vi "Update Steps LEDs.vi"(8 "error in":errorcluster, 10 "Wash Steps Selected":T1(array[cluster]), 11 "Car Wash Indicators Ref":refnum<vi>) -> (0 "error out":errorcluster)   [LabVIEW 2020]
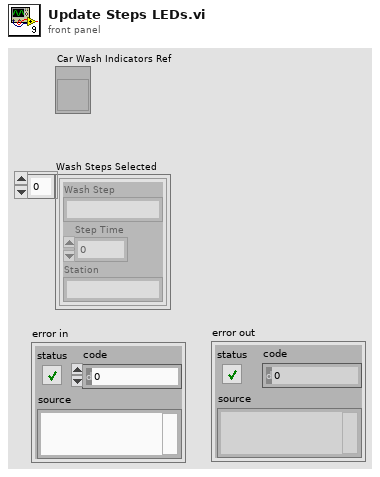
[diagram p1: front panel]
types:
  T1 = cluster{"Wash Step":string, "Step Time":i32, "Station":string}[]
  T2 = cluster{"Wash Step":string, "Step Time":i32, "Station":string}
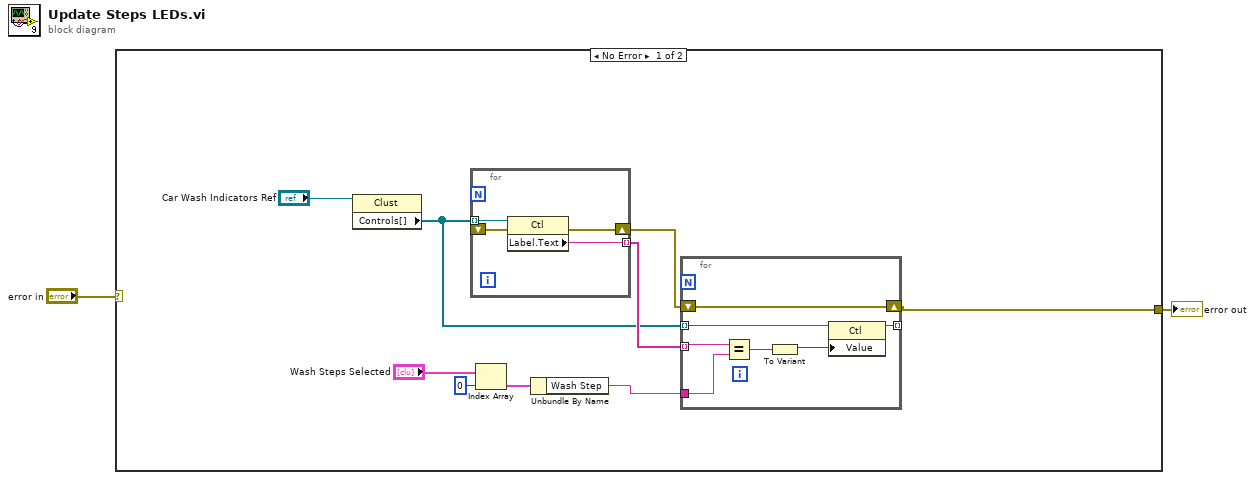
[diagram p0: block diagram]
diagram:
  n1 = case shown="No Error" "error in" {
    selector: "error in" -> [_ w23]
    tunnel: [w3 w23] -> w2
    frame No Error {
      n2 = property class="Clust"(reference="Car Wash Indicators Ref") -> ("Controls[]"=w5:refnum<vi>[])  [unwired: 1 in, 2 out]
      n3 = for {
        tunnel: w5 -> [w22] mode=indexing
        tunnel: [w21] -> w7 mode=indexing
        shift-right: [w20] -> w6
        shift-left: _ -> [w19]
        n4 = property class="Ctl"(reference=w22, error in=w19) -> (error out=w20:errorcluster, "Label.Text"=w21:string)  [unwired: 1 out]
      }
      n5 = Index Array(array="Wash Steps Selected", index=0) -> (element=w10:T2)
      n6 = Unbundle By Name(w10) -> ("Wash Step"=w11:string)
      n7 = for {
        tunnel: w5 -> [w18] mode=indexing
        tunnel: w7 -> [w17] mode=indexing
        tunnel: w11 -> [w16]
        tunnel: [w13] -> _ mode=indexing
        shift-right: [w12] -> w3
        shift-left: w6 -> [w12]
        n8 = Equal?(x=w17, y=w16) -> (x = y?=w15:bool)
        n9 = To Variant(anything=w15) -> (Variant=w14:variant)
        n10 = property class="Ctl"(reference=w18, "Value"=w14) -> (reference out=w13:refnum<vi>)  [unwired: 1 in, 1 out]
      }
    }
    frame Error {
    }
  }
  "error out" <- w2
